vi "Set_Traverse_Position.vi"(3 "Last Part of Move?":bool=TRUE, 4 "Currently on Point":i32=11, 5 "Simulate/Run":T3, 6 "Traverse line":T4 {"Carrier_2 Q (l/min)" format="%#.2f"; "Row Duration (mins)" format="%#.1f"; "Row No" min=0; "Trace Gas Concentration (%)" min=0.0 format="%#_4f"; "Carrier_1 Q (l/min)" format="%#.2f"; "Tunnel Speed" format="%#.2f"; "Start X" format="%#.2f"; "Start Y" format="%#.2f"; "Start Z" format="%#.2f"; "End X" format="%#.2f"; "End Y" format="%#.2f"; "End Z" format="%#.2f"; "Averaging time (min)" min=0.0 format="%#.2f"}) -> (0 "Status Cluster":T1)   [LabVIEW 2014]
uses:
  Traverse_cluster.ctl
  Spacing.ctl
  Controls/Multi_run_mode.ctl
  Controls/User_Specific_mode.ctl
  Status_Cluster.ctl
  Multi_Run_Status.ctl
  Trav_mode.ctl
  Controls/Home.ctl
  Globals/Extra_Commands_Global.vi
  Globals/Dynamic_call_global.ph.vi
  Globals/Constants_global.vi
panel:
  # "X           Y            Z"
  # "Start"
  # "End"
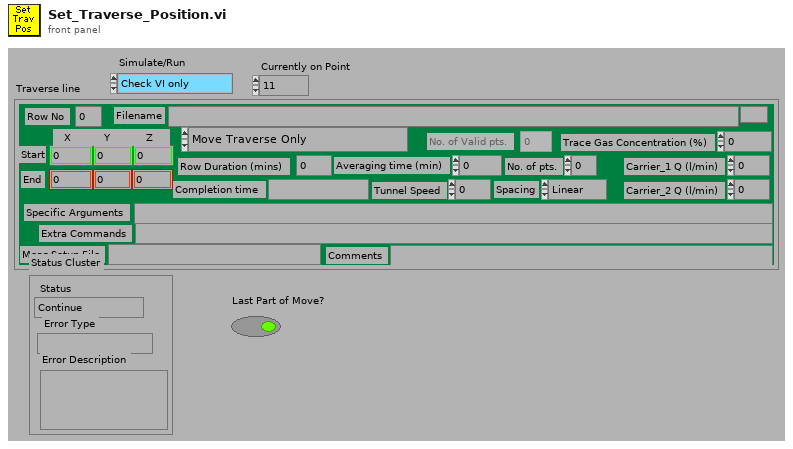
[diagram p1: front panel]
types:
  T1 = typedef "Status_Cluster.ctl" = cluster{"Status":T2, "Error Type":string, "Error Description":string}
  T2 = typedef "Multi_Run_Status.ctl" = enum16{"Continue", "Jump to Next Point", "Jump to Next Row", "Jump To Fall Back", "Terminate Run"}
  T3 = typedef "User_Specific_mode.ctl" = enum16{"Check VI only", "Run VI"}
  T4 = typedef "Traverse_cluster.ctl" = cluster{"Start X":sgl, "Start Y":sgl, "Start Z":sgl, "End X":sgl, "End Y":sgl, "End Z":sgl, "No. of pts.":i32, "Spacing":T5, "Filename":path, "Tunnel Speed":dbl, "Averaging time (min)":dbl, "Extra Commands":string, "Carrier_1 Q (l/min)":dbl, "Carrier_2 Q (l/min)":dbl, "Trace Gas Concentration (%)":dbl, "Specific Arguments":string, "Comments":string, "Row No":i32, "Row Type Selector":T6, "Completion time":string, "Row Duration (mins)":dbl, "No. of Valid pts.":i32, "Meas Setup File":string}
  T5 = typedef "Spacing.ctl" = enum16{"Linear", "Log", "Gauss", "Specified", "N/A"}
  T6 = typedef "Multi_run_mode.ctl" = enum16{"Move Traverse Only", "Set Tunnel Speed Only", "Set Source Only", "Set Measurement Conditions", "Single Measurement", "Vertical Profile", "Lateral Profile", "Longitudinal Profile", "Explore Volume", "Multi-Axis Profile", "Auto Calibrate", "Meas Fast FID Bkgnd", "Check Beam Power", "Scanning Valve Measurement", "Run VI Named:", "Set ADAM Ch", "Wait (minutes)", "Send Message", "Synchronize With:", "Fall Back to this Row", "Turn Off Row Repeating", "Blank Row", "Traverse 3D Volume"}
  T7 = typedef "Trav_mode.ctl" = enum16{"Move traverse", "Read traverse position", "Teach Position"}
  T8 = typedef "Home.ctl" = enum16{"Don't Home", "Home  +X", "Home  -X", "Home  +Y", "Home  -Y", "Home  +Z", "Home  -Z"}
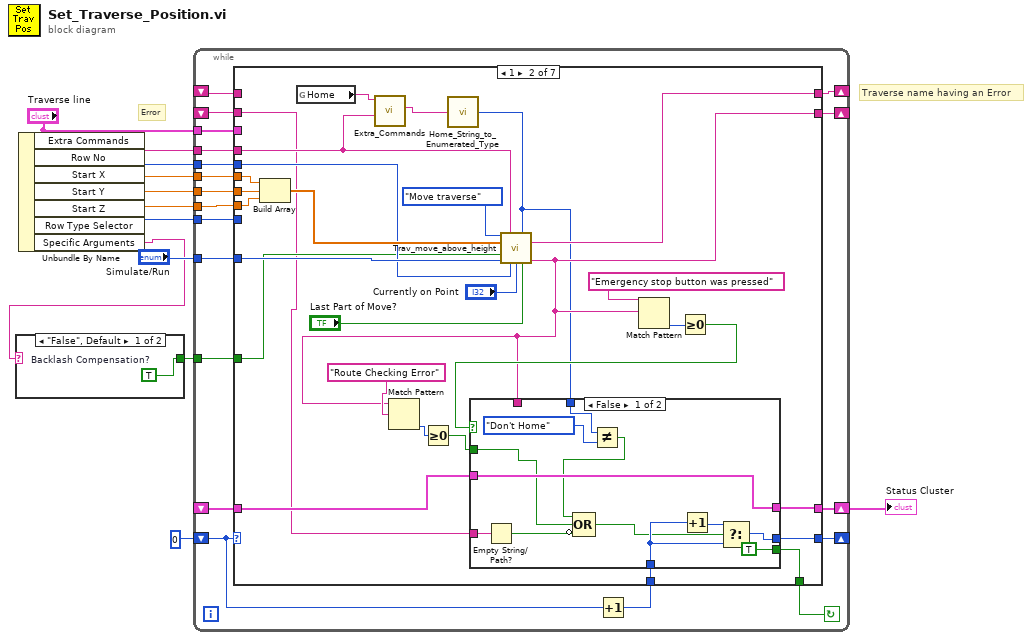
[diagram p0: block diagram]
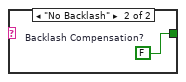
[diagram p2: hidden frame]
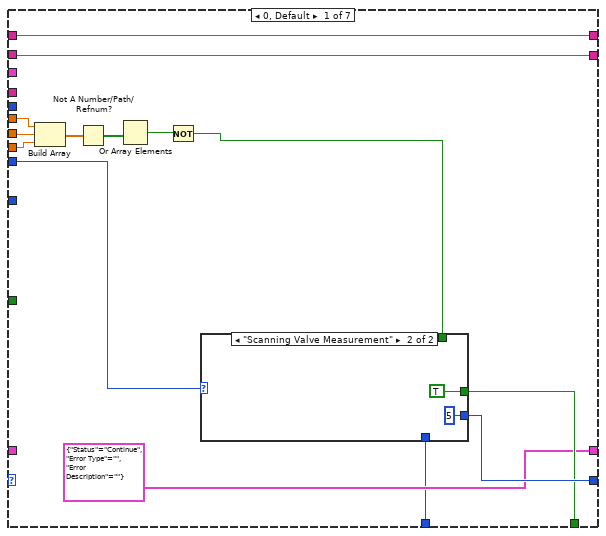
[diagram p3: hidden frame]
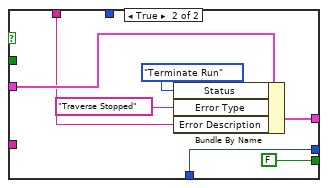
[diagram p5: hidden frame]
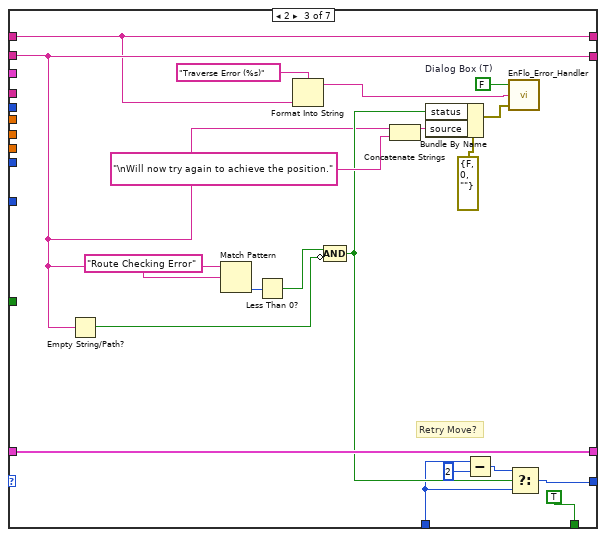
[diagram p6: hidden frame]
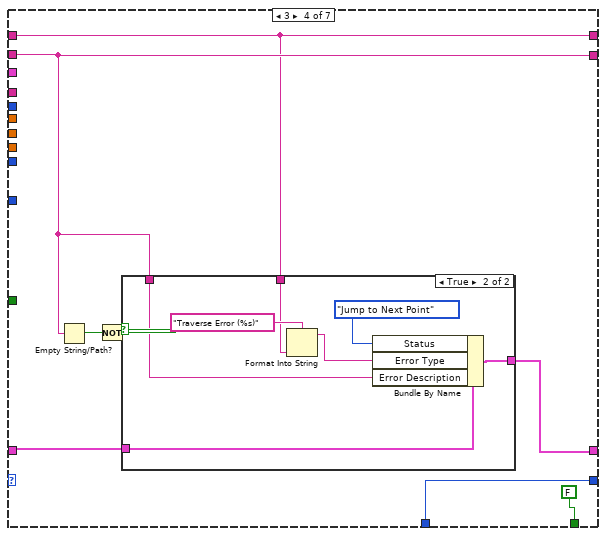
[diagram p7: hidden frame]
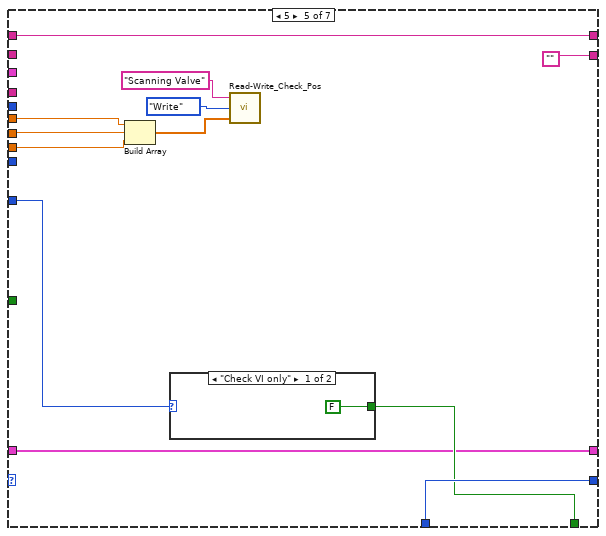
[diagram p9: hidden frame]
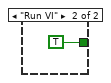
[diagram p10: hidden frame]
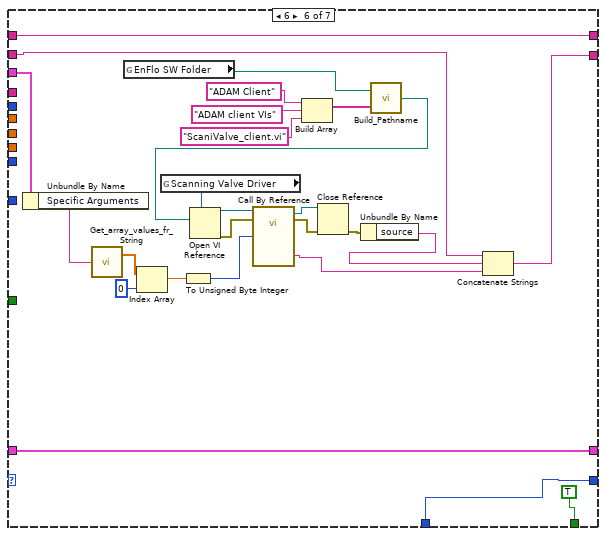
[diagram p11: hidden frame]
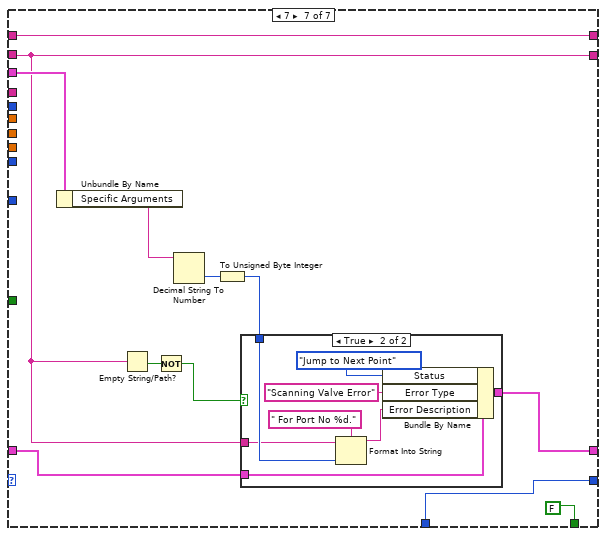
[diagram p12: hidden frame]
diagram:
  # "Traverse name having an Error"
  # "Error"
  n1 = Unbundle By Name("Traverse line") -> ("Extra Commands"=w11:string, "Row No"=w10:i32, "Start X"=w7:sgl, "Start Y"=w12:sgl, "Start Z"=w6:sgl, "Row Type Selector"=w8:T6, "Specific Arguments"=w2:string)
  n2 = case shown="\"False\", Default" w2 {
    tunnel: [w13 w14] -> w1
    frame "False", Default {
      w13 = TRUE  # Backlash Compensation?
    }
    frame "No Backlash" {
      w14 = FALSE  # Backlash Compensation?
    }
  }
  n3 = while {
    shift-left: _ -> [w18]
    shift-right: [w19] -> _
    shift-left: _ -> [w20]
    shift-right: [w21] -> w3
    tunnel: "Traverse line" -> [w22]
    tunnel: "Simulate/Run" -> [w23]
    tunnel: w6 -> [w24]
    tunnel: w12 -> [w25]
    tunnel: w7 -> [w26]
    tunnel: w8 -> [w31]
    shift-left: 0 -> [w29]
    shift-right: [w28] -> _
    tunnel: w10 -> [w32]
    tunnel: w11 -> [w33]
    tunnel: w1 -> [w17]
    shift-right: [w16] -> _
    shift-left: _ -> [w15]
    stop <- w30 continue-if-true
    n4 = Increment(x=w29) -> (x+1=w27:i32)
    n5 = case shown="1" w29 {
      tunnel: w33 -> [_ w57 _ _ _ _ _]
      tunnel: w32 -> [_ w70 _ _ _ _ _]
      tunnel: w31 -> [w47 _ _ _ _ _ _]
      tunnel: [w45 w64 TRUE FALSE w144 TRUE FALSE] -> w30
      tunnel: [w46 w71 w104 w124 w146 w151 w176] -> w28
      tunnel: w27 -> [w43 w72 w105 w124 w146 w151 w176]
      tunnel: w26 -> [w39 w77 _ _ w138 _ _]
      tunnel: w25 -> [w40 w76 _ _ w137 _ _]
      tunnel: w24 -> [w41 w75 _ _ w136 _ _]
      tunnel: w23 -> [_ w73 _ _ w145 _ _]
      tunnel: w22 -> [_ _ _ _ _ w168 w185]
      tunnel: [T1 {"Status"=enum."Continue", "Error Type"="", "Error Description"=""} ("Status Cluster") w66 w113 w125 w143 w159 w182] -> w21
      tunnel: w20 -> [_ w65 w113 w126 w143 w159 w183]
      tunnel: [w42 w62 w103 w121 "" w152 w177] -> w19
      tunnel: w18 -> [w42 w56 w103 w121 _ w150 w177]
      tunnel: w17 -> [_ w59 _ _ _ _ _]
      tunnel: [w34 w58 w99 w119 w135 w149 w175] -> w16
      tunnel: w15 -> [w34 _ w99 w119 w135 w149 w175]
      frame 0, Default {
        n6 = Build Array(w39, w40, w41) -> (w38:sgl[])
        n7 = Not A Number/Path/Refnum?(number/path/refnum=w38) -> (NaN/Path/Refnum?=w37:bool[])
        n8 = Or Array Elements(Boolean array=w37) -> (logical OR=w36:bool)
        n9 = Not(x=w36) -> (.not. x?=w35:bool)
        n10 = case shown="\"Scanning Valve Measurement\"" w47 {
          tunnel: [w48 5] -> w46
          tunnel: [w49 TRUE] -> w45
          tunnel: w35 -> [w49 _]
          tunnel: w43 -> [w48 _]
          frame "Move Traverse Only", Default {
          }
          frame "Scanning Valve Measurement" {
          }
        }
      }
      frame 1 {
        n11 = Build Array(w77, w76, w75) -> (w74:sgl[])
        n12 = global read "Extra_Commands_Global.vi" "Home"() -> (w55:string)
        n13 = call "Extra_Commands.vi"("String to Search"=w57, "Command"=w55) -> ("String Value"=w54:string)  [unwired: 1 in, 4 out]
        n14 = call "Home_String_to_Enumerated_Type.vi"("String"=w54) -> ("Home"=w53:T8)
        n15 = call "Trav_move_above_height.vi"("Mode"=Trav_mode."Move traverse", "Extra Command String"=w57, "Home Z"=w53, "New Position"=w74, "Backlash Compensation?"=w59, "Simulate/Run"=w73, "Row Number"=w70, "Currently on Point"="Currently on Point", "Last Part of Move?"="Last Part of Move?") -> ("Error from Traverse named"=w58:string, "Error String"=w62:string)  [unwired: 4 in, 1 out]
        n16 = Match Pattern(string=w62, regular expression="Route Checking Error") -> (offset past match=w61:i32)  [unwired: 4 out]
        n17 = Greater Or Equal To 0?(x=w61) -> (x >= 0?=w60:bool)
        n18 = Match Pattern(string=w62, regular expression="Emergency stop button was pressed") -> (offset past match=w68:i32)  [unwired: 4 out]
        n19 = Greater Or Equal To 0?(x=w68) -> (x >= 0?=w67:bool)
        n20 = case shown="False" w67 {
          tunnel: w72 -> [w90 w93]
          tunnel: [w89 w93] -> w71
          tunnel: w56 -> [w88 _]
          tunnel: [w87 w95] -> w66
          tunnel: w65 -> [w87 w96]
          tunnel: w62 -> [_ w94]
          tunnel: [TRUE FALSE] -> w64
          tunnel: w60 -> [w85 _]
          tunnel: w53 -> [w82 _]
          frame False {
            n21 = Empty String/Path?(string/path=w88) -> (empty?=w83:bool)
            n22 = Not Equal?(x=w82, y=Home."Don't Home" ("Home")) -> (x != y?=w80:bool)
            n23 = Compound Arithmetic op=OR(w80, w85, invert w83) -> (w84:bool)
            n24 = Increment(x=w90) -> (x+1=w91:i32)
            n25 = Select(t=w91, s=w84, f=w90) -> (s? t:f=w89:i32)
          }
          frame True {
            n26 = Bundle By Name(cluster=w96, "Status"=Multi_Run_Status."Terminate Run", "Error Type"="Traverse Stopped" ("t"), "Error Description"=w94) -> (w95:T1)
          }
        }
      }
      frame 2 {
        w116 = FALSE  # Dialog Box (T)
        # "Retry Move?"
        n27 = Empty String/Path?(string/path=w103) -> (empty?=w102:bool)
        n28 = Match Pattern(string=w103, regular expression="Route Checking Error" ("String to match")) -> (offset past match=w110:i32)  [unwired: 4 out]
        n29 = Less Than 0?(x=w110) -> (x < 0?=w109:bool)
        n30 = Format Into String(format string="Traverse Error (%s)" ("t"), w99) -> (resulting string=w100:string)  [unwired: 2 in, 1 out]
        n31 = Compound Arithmetic op=AND(w109, invert w102) -> (w108:bool)
        n32 = Concatenate Strings(w103, "\nWill now try again to achieve the position." ("Substring")) -> (w115:string)
        n33 = Bundle By Name(cluster=errorcluster {"status"=FALSE, "code"=0, "source"=""} ("error in (no error)"), "status"=w108, "source"=w115) -> (w117:errorcluster)
        n34 = Subtract(x=w105, y=2) -> (x-y=w106:i32)
        n35 = call "EnFlo_Error_Handler.vi"("error in (no error)"=w117, "Error Type"=w100, "Dialog Box (T)"=w116) -> ()  [unwired: 3 out]
        n36 = Select(t=w106, s=w108, f=w105) -> (s? t:f=w104:i32)
      }
      frame 3 {
        n37 = Empty String/Path?(string/path=w121) -> (empty?=w122:bool)
        n38 = Not(x=w122) -> (.not. x?=w120:bool)
        n39 = case shown="True" w120 {
          tunnel: w126 -> [w127 w134]
          tunnel: [w127 w132] -> w125
          tunnel: w121 -> [_ w131]
          tunnel: w119 -> [_ w128]
          frame False {
          }
          frame True {
            n40 = Format Into String(format string="Traverse Error (%s)" ("t"), w128) -> (resulting string=w129:string)  [unwired: 2 in, 1 out]
            n41 = Bundle By Name(cluster=w134, "Status"=Multi_Run_Status."Jump to Next Point", "Error Type"=w129, "Error Description"=w131) -> (w132:T1)
          }
        }
      }
      frame 5 {
        n42 = Build Array(w138, w137, w136) -> (w141:sgl[])
        n43 = case shown="\"Check VI only\"" w145 {
          tunnel: [FALSE TRUE] -> w144
          frame "Check VI only" {
          }
          frame "Run VI" {
          }
        }
        n44 = call "Read-Write_Check_Pos.vi"("Position input"=w141, "Mode"=enum16{"Read", "Write"}."Write", "Traverse Name"="Scanning Valve") -> ()  [unwired: 1 out]
      }
      frame 6 {
        n45 = Unbundle By Name(w168) -> ("Specific Arguments"=w156:string)
        n46 = call "Get_array_values_fr_String.vi"("String Value"=w156) -> ("Numeric Array"=w158:dbl[])  [unwired: 1 out]
        n47 = global read "Constants_global.vi" "EnFlo SW Folder"() -> (w162:path)
        n48 = Index Array(array=w158, index=0) -> (element=w155:dbl)
        n49 = global read "Dynamic_call_global.ph.vi" "Scanning Valve Driver"() -> (w169:refnum<vi>)
        n50 = To Unsigned Byte Integer(number=w155) -> (unsigned 8bit integer=w167:u8)
        n51 = Build Array("ADAM Client", "ADAM client VIs", "ScaniValve_client.vi") -> (w163:string[])
        n52 = call "Build_Pathname.vi"("PathElements"=w163, "PathnameIn"=w162) -> ("AppendedPath"=w161:path)
        n53 = Open VI Reference(type specifier VI Refnum (for type only)=w169, vi path=w161) -> (vi reference=w170:refnum<vi>, error out=w171:errorcluster)  [unwired: 2 in, 2 out]
        n54 = call-by-ref "?"(reference=w170, error in=w171, "Port Number"=w167) -> (reference out=w173:refnum<vi>, error out=w172:errorcluster, "Error String"=w153:string)  [unwired: 2 out]
        n55 = Close Reference(reference=w173, error in (no error)=w172) -> (error out=w174:errorcluster)
        n56 = Unbundle By Name(w174) -> ("source"=w154:string)
        n57 = Concatenate Strings(w150, w154, w153) -> (w152:string)
      }
      frame 7 {
        n58 = Unbundle By Name(w185) -> ("Specific Arguments"=w186:string)
        n59 = Empty String/Path?(string/path=w177) -> (empty?=w179:bool)
        n60 = Not(x=w179) -> (.not. x?=w178:bool)
        n61 = Decimal String To Number(string=w186) -> (number=w184:i32)  [unwired: 3 out]
        n62 = To Unsigned Byte Integer(number=w184) -> (unsigned 8bit integer=w181:u8)
        n63 = case shown="True" w178 {
          tunnel: w183 -> [w187 w195]
          tunnel: [w187 w192] -> w182
          tunnel: w181 -> [_ w190]
          tunnel: w177 -> [_ w188]
          frame False {
          }
          frame True {
            n64 = Format Into String(format string=" For Port No %d." ("Format String"), initial string=w188, w190) -> (resulting string=w189:string)  [unwired: 1 in, 1 out]
            n65 = Bundle By Name(cluster=w195, "Status"=Multi_Run_Status."Jump to Next Point", "Error Type"="Scanning Valve Error" ("t"), "Error Description"=w189) -> (w192:T1)
          }
        }
      }
    }
  }
  "Status Cluster" <- w3
